vi "Encoding--constant.vi"() -> (3 "Encoding (none)":string)   [LabVIEW 2020]
doc: "Encoding of XML Cache file."
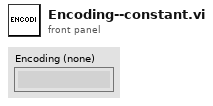
[diagram p1: front panel]
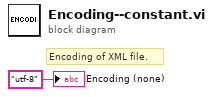
[diagram p0: block diagram]
diagram:
  # "Encoding of XML file."
  "Encoding (none)" <- "utf-8" ("Encoding (none)")
